vi "Trim Whitespace.vi"(1 "Input":string) -> (0 "Output":string)   [LabVIEW 2020, in "ase.lvlib" / "ase.lvclass"]
doc: "Trim whitespace characters from the front and back of a string."
uses:
  ase.lvclass
  ase.lvclass/ase.ctl
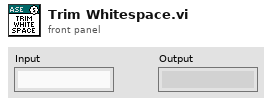
[diagram p1: front panel]
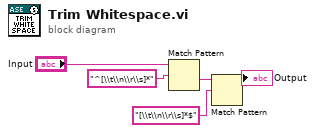
[diagram p0: block diagram]
diagram:
  n1 = Match Pattern(string="Input", regular expression="^[\\t\\n\\r\\s]*") -> (after substring=w3:string)  [unwired: 1 in, 3 out]
  n2 = Match Pattern(string=w3, regular expression="[\\t\\n\\r\\s]*$") -> (before substring=→"Output":string)  [unwired: 1 in, 3 out]
